vi "Tank Fill.vi"() -> ()   [LabVIEW 2013]
uses:
  Tank Fill Global.vi
panel:
  in  "Stop Fill":bool
  in  "Start Fill":bool
  out "Bottom Float Switch":bool
  out "Top Float Switch":bool
  out "Tank level":i32(slide) scale=0.0..300.0
  # "Click          to run"
  # "Tank Fill"
  # "Here, there is a 300 gallon mix tank which mixes red dye.  It drains at a constant rate of 50 gal/sec. There is a pump that can add dye at a rate of 100 gal/sec.\nThere are two float switches, which monitor the level in the tank. When the dye level reaches one of the switches, it is activated, and its value becomes true.\n\nYour job is to add this functionality:\nThe pump is activated by the Start Fill button. When this starts, dye gets pumped into the mix tank until it hits the top float switch. Once this switch is reached, the pump turns off.  \nThe tank level decreases until it the level goes below the bottom float switch. At this point, the pump should start back up and restart the cycle. The tank level should oscillate between the two float switches like this until the stop fill button is pushed, at which point the tank will drain."
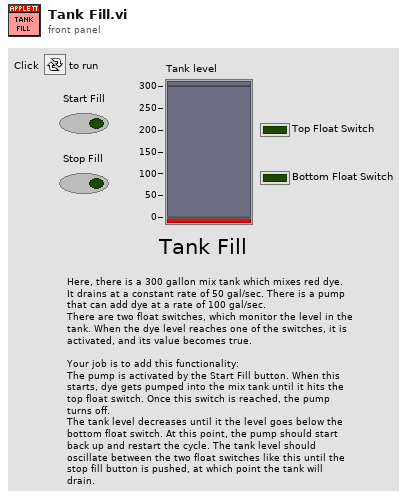
[diagram p1: front panel]
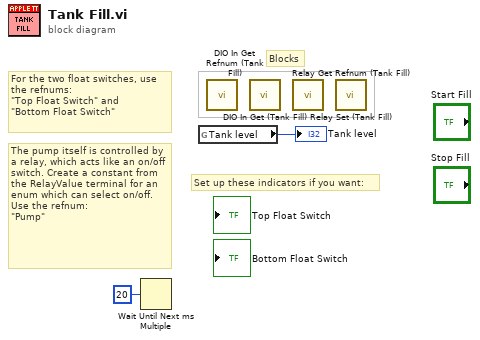
[diagram p0: block diagram]
diagram:
  # "The pump itself is controlled by a relay, which acts like an on/off switch. Create a constant from the RelayValue terminal for an enum which can select on/off.\nUse the refnum:\n\"Pump\""
  # "For the two float switches, use\nthe refnums:\n\"Top Float Switch\" and\n\"Bottom Float Switch\""
  # "Set up these indicators if you want:"
  # "Blocks"
  n1 = Wait Until Next ms Multiple(millisecond multiple=u32 20) -> ()  [unwired: 1 out]
  n2 = global read "Tank Fill Global.vi" "Tank level"() -> (→"Tank level":i32)
  n3 = call "DIO In Get Refnum (Tank Fill).vi"() -> ()  [unwired: 10 in, 2 out]
  n4 = call "DIO In Get (Tank Fill).vi"() -> ()  [unwired: 9 in, 3 out]
  n5 = call "Relay Get Refnum (Tank Fill).vi"() -> ()  [unwired: 10 in, 2 out]
  n6 = call "Relay Set (Tank Fill).vi"() -> ()  [unwired: 10 in, 2 out]
